vi "Store Config.vi"(8 "error in":errorcluster, 11 "Philips UI in":refnum<class "Flex UI.lvclass">) -> (0 "error out":errorcluster, 3 "Philips UI out":refnum<class "Flex UI.lvclass">)   [LabVIEW 2014, in "Flex UI.lvclass"]
uses:
  Flex UI.lvclass
  Flex UI.lvclass/Flex UI.ctl
  <vilib>/Utility/config.llb/NI_LVConfig.lvlib
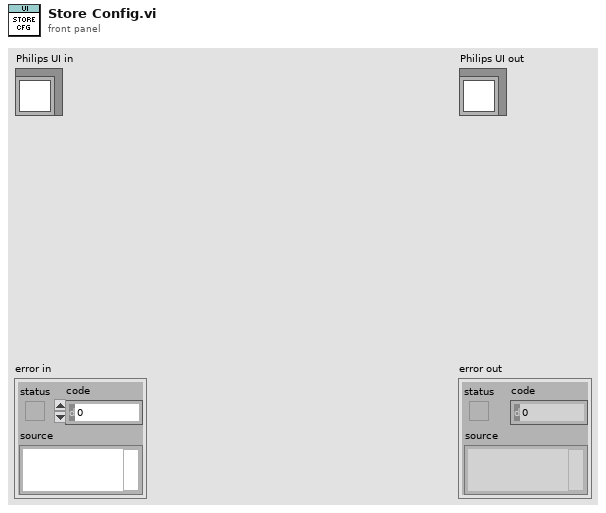
[diagram p1: front panel]
types:
  T1 = typedef "NI_LVConfig.lvlib/Config Data RefNum.ctl" = refnum<k1>
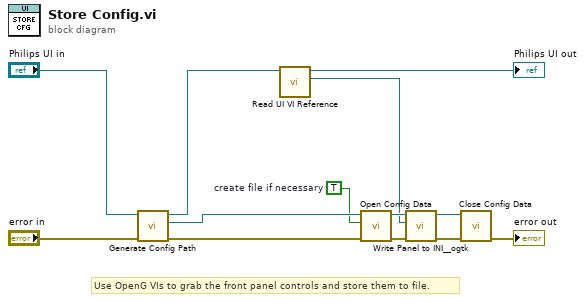
[diagram p0: block diagram]
diagram:
  w1 = TRUE  # create file if necessary
  # "Use OpenG VIs to grab the front panel controls and store them to file."
  n1 = call-dynamic "Generate Config Path.vi"("error in"="error in", "Philips UI in"="Philips UI in") -> ("error out"=w6:errorcluster, "Config Path"=w2:path, "Philips UI out"=w4:refnum<class "Flex UI.lvclass">)  [unwired: 7 in]
  n2 = call "Read UI VI Reference.vi"("Philips UI in"=w4) -> ("UI VI Reference"=w7:refnum<vi>, "Philips UI out"=→"Philips UI out":refnum<class "Flex UI.lvclass">)  [unwired: 9 in]
  n3 = call <vilib>:"Open Config Data.vi"("error in (no error)"=w6, "create file if necessary (T)"=w1, "configuration file path"=w2) -> ("error out"=w11:errorcluster, "refnum"=w10:T1)  [unwired: 6 in, 1 out]
  n4 = call <userlib>:"Write Panel to INI__ogtk.vi"("error in (no error)"=w11, "VI ref"=w7, "refnum"=w10) -> ("error out"=w12:errorcluster, "refnum out"=w13:T1)  [unwired: 7 in]
  n5 = call <vilib>:"Close Config Data.vi"("error in (no error)"=w12, "refnum"=w13) -> ("error out"=→"error out":errorcluster)  [unwired: 8 in, 1 out]
